vi "Lars.vi"(8 "error in":errorcluster) -> (0 "error out":errorcluster, 3 "out":refnum<class "Lars.lvclass">)   [LabVIEW 2020]
doc: "Least Angle Regression model a.k.a. LAR\n\n Read more in the :ref:`User Guide <least_angle_regression>`.\n\n Parameters\n ----------\n fit_intercept : bool, default=True\n Whether to calculate the intercept for this model. If set\n to false, no intercept will be used in calculations\n (i.e. data is expected to be centered).\n\n verbose : bool or int, default=False\n Sets the verbosity amount.\n\n normalize : bool, default=True\n This parameter is ignored when ``fit_intercept`` is set to False.\n If True, the regressors X will be normalized before regression by\n subtracting the mean and dividing by the l2-norm.\n If you wish to standardize, please use\n :class:`~sklearn.preprocessing.StandardScaler` before calling ``fit``\n on an estimator with ``normalize=False``.\n\n precompute : bool, 'auto' or array-like , default='auto'\n Whether to use a precomputed Gram matrix to speed up\n calculations. If set to ``'auto'`` let us decide. The Gram\n matrix can also be passed as argument.\n\n n_nonzero_coefs : int, default=500\n Target number of non-zero coefficients. Use ``np.inf`` for no limit.\n\n eps : float, default=np.finfo(float).eps\n The machine-precision regularization in the computation of the\n Cholesky diagonal factors. Increase this for very ill-conditioned\n systems. Unlike the ``tol`` parameter in some iterative\n optimization-based algorithms, this parameter does not control\n the tolerance of the optimization.\n\n copy_X : bool, default=True\n If ``True``, X will be copied; else, it may be overwritten.\n\n fit_path : bool, default=True\n If True the full path is stored in the ``coef_path_`` attribute.\n If you compute the solution for a large problem or many targets,\n setting ``fit_path`` to ``False`` will lead to a speedup, especially\n with a small alpha.\n\n jitter : float, default=None\n Upper bound on a uniform noise parameter to be added to the\n `y` values, to satisfy the model's assumption of\n one-at-a-time computations. Might help with stability.\n\n .. versionadded:: 0.23\n\n random_state : int, RandomState instance or None, default=None\n Determines random number generation for jittering. Pass an int\n for reproducible output across multiple function calls.\n See :term:`Glossary <random_state>`. Ignored if `jitter` is None.\n\n .. versionadded:: 0.23\n\n Attributes\n ----------\n alphas_ : array-like of shape (n_alphas + 1,) or list of such arrays\n Maximum of covariances (in absolute value) at each iteration.\n ``n_alphas`` is either ``max_iter``, ``n_features`` or the\n number of nodes in the path with ``alpha >= alpha_min``, whichever\n is smaller. If this is a list of array-like, the length of the outer\n list is `n_targets`.\n\n active_ : list of shape (n_alphas,) or list of such lists\n Indices of active variables at the end of the path.\n If this is a list of list, the length of the outer list is `n_targets`.\n\n coef_path_ : array-like of shape (n_features, n_alphas + 1) or list of such arrays\n The varying values of the coefficients along the path. It is not\n present if the ``fit_path`` parameter is ``False``. If this is a list\n of array-like, the length of the outer list is `n_targets`.\n\n coef_ : array-like of shape (n_features,) or (n_targets, n_features)\n Parameter vector (w in the formulation formula).\n\n intercept_ : float or array-like of shape (n_targets,)\n Independent term in decision function.\n\n n_iter_ : array-like or int\n The number of iterations taken by lars_path to find the\n grid of alphas for each target.\n\n \nAvailable methods:\nGet Attributes\nGet Params\nSet Params"
uses:
  Lars.lvclass
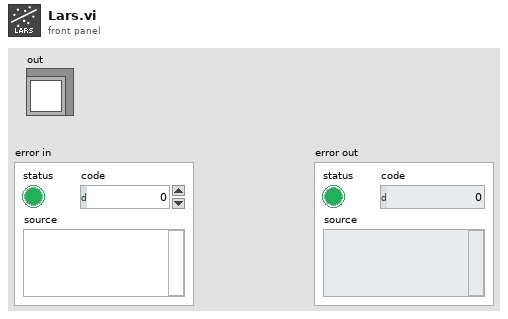
[diagram p1: front panel]
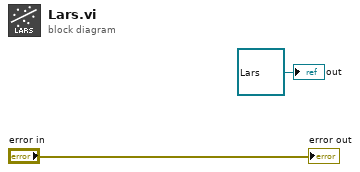
[diagram p0: block diagram]
diagram:
  "out" <- refnum<class "Lars.lvclass"> refnum ("model")
  "error out" <- "error in"
